vi "Get Connection id.vi"(11 "Reply Protocol DataSocket in":refnum<class "Reply Protocol DataSocket.lvclass">) -> (2 "Connection id":refnum<k13>, 3 "Reply Protocol DataSocket out":refnum<class "Reply Protocol DataSocket.lvclass">)   [LabVIEW 2023, in "HAL GOOP4.lvlib" / "Reply Protocol DataSocket.lvclass"]
uses:
  Reply Protocol DataSocket.lvclass
  Reply Protocol DataSocket.lvclass/Reply Protocol DataSocket.ctl
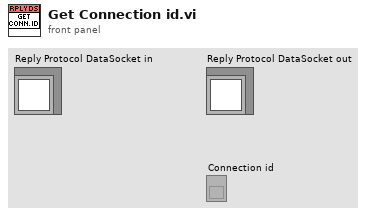
[diagram p1: front panel]
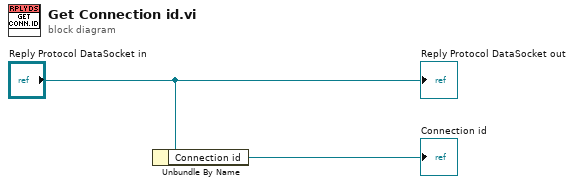
[diagram p0: block diagram]
diagram:
  n1 = Unbundle By Name("Reply Protocol DataSocket in") -> ("Connection id"=→"Connection id":refnum<k13>)
  "Reply Protocol DataSocket out" <- "Reply Protocol DataSocket in"
